vi "Emerson 5700 Basic Tester.vi"(8 "Error In":errorcluster, 11 "Remote IP Address":string="10.2.0.49") -> (0 "Error Out":errorcluster, 3 "Emerson Flow Meter Data Output":T1)   [LabVIEW 2016]
uses:
  Type Definitions/Emerson 5700 Data.ctl
  <vilib>/NI/Modbus Library/API/Wrapper/Create TCP Master.vi
  <vilib>/NI/Modbus Library/API/Master/Modbus Master.lvclass
  <vilib>/NI/Modbus Library/API/Wrapper/API Main.lvlib
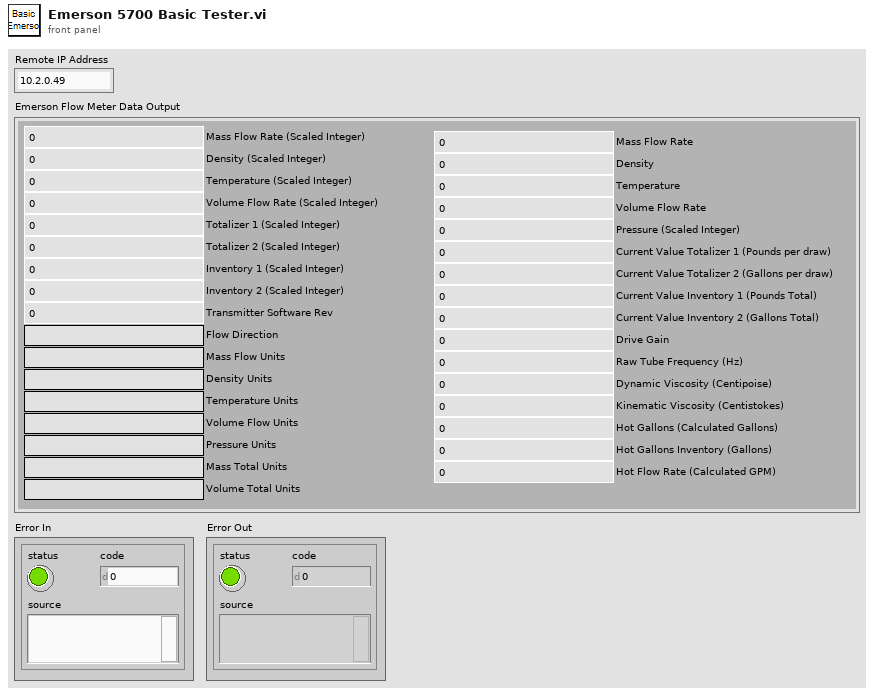
[diagram p1: front panel]
types:
  T1 = typedef "Emerson 5700 Data.ctl" = cluster{"Mass Flow Rate (Scaled Integer)":u16, "Density (Scaled Integer)":u16, "Temperature (Scaled Integer)":u16, "Volume Flow Rate (Scaled Integer)":u16, "Totalizer 1 (Scaled Integer)":u16, "Totalizer 2 (Scaled Integer)":u16, "Transmitter Software Rev":u16, "Flow Direction":string, "Mass Flow Units":string, "Density Units":string, "Temperature Units":string, "Volume Flow Units":string, "Pressure Units":string, "Mass Total Units":string, "Volume Total Units":string, "Inventory 1 (Scaled Integer)":u16, "Inventory 2 (Scaled Integer)":u16, "Mass Flow Rate":dbl, "Density":dbl, "Temperature":dbl, "Volume Flow Rate":dbl, "Pressure (Scaled Integer)":u16, "Current Value Totalizer 1 (Pounds per draw)":dbl, "Current Value Totalizer 2 (Gallons per draw)":dbl, "Current Value Inventory 1 (Pounds Total)":dbl, "Current Value Inventory 2 (Gallons Total)":dbl, "Drive Gain":dbl, "Raw Tube Frequency (Hz)":dbl, "Dynamic Viscosity (Centipoise)":dbl, "Kinematic Viscosity (Centistokes)":dbl, "Hot Gallons (Calculated Gallons)":dbl, "Hot Flow Rate (Calculated GPM)":dbl, "Hot Gallons Inventory (Gallons)":dbl}
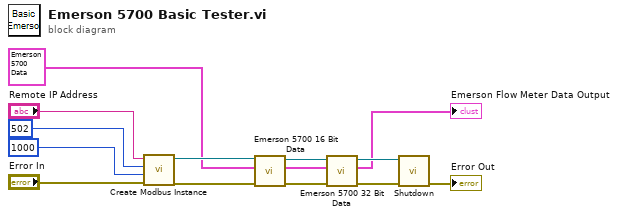
[diagram p0: block diagram]
diagram:
  n1 = call-poly <vilib>:"Create Modbus Instance.vi"("error in"="Error In", "connect timeout ms"=1000, "port (502)"=u16 502, "address"="Remote IP Address") -> ("error out"=w12:errorcluster, "TCP master instance"=w11:refnum<class "Modbus Master.lvclass">)  [unwired: 6 in]
  n2 = call "Emerson 5700 16 Bit Data.vi"("error in (no error)"=w12, "Emerson Flow Meter Data Input"=T1 {"Mass Flow Rate (Scaled Integer)"=0, "Density (Scaled Integer)"=0, "Temperature (Scaled Integer)"=0, "Volume Flow Rate (Scaled Integer)"=0, "Totalizer 1 (Scaled Integer)"=0, "Totalizer 2 (Scaled Integer)"=0, "Transmitter Software Rev"=0, "Flow Direction"="", "Mass Flow Units"="", "Density Units"="", "Temperature Units"="", "Volume Flow Units"="", "Pressure Units"="", "Mass Total Units"="", "Volume Total Units"="", "Inventory 1 (Scaled Integer)"=0, "Inventory 2 (Scaled Integer)"=0, "Mass Flow Rate"=0.0, "Density"=0.0, "Temperature"=0.0, "Volume Flow Rate"=0.0, "Pressure (Scaled Integer)"=0, "Current Value Totalizer 1 (Pounds per draw)"=0.0, "Current Value Totalizer 2 (Gallons per draw)"=0.0, "Current Value Inventory 1 (Pounds Total)"=0.0, "Current Value Inventory 2 (Gallons Total)"=0.0, "Drive Gain"=0.0, "Raw Tube Frequency (Hz)"=0.0, "Dynamic Viscosity (Centipoise)"=0.0, "Kinematic Viscosity (Centistokes)"=0.0, "Hot Gallons (Calculated Gallons)"=0.0, "Hot Flow Rate (Calculated GPM)"=0.0, "Hot Gallons Inventory (Gallons)"=0.0}, "Modbus Master in"=w11) -> ("error out"=w9:errorcluster, "Emerson Flow Meter Data Output"=w5:T1, "Modbus Master out"=w8:refnum<class "Modbus Master.lvclass">)  [unwired: 6 in]
  n3 = call "Emerson 5700 32 Bit Data.vi"("Error In"=w9, "Emerson Flow Meter Data Input"=w5, "Modbus master in"=w8) -> ("Error Out"=w7:errorcluster, "Emerson Flow Meter Data Output"=→"Emerson Flow Meter Data Output":T1, "Modbus master out"=w6:refnum<class "Modbus Master.lvclass">)  [unwired: 6 in]
  n4 = call-dynamic "Shutdown.vi"("error in"=w7, "Modbus master in"=w6) -> ("error out"=→"Error Out":errorcluster)  [unwired: 9 in]
